vi "Example Circular Buffer Map.vi"() -> ()   [LabVIEW 2013]
uses:
  VariantBuffer/VariantBuffer.lvclass
  VariantBufferMap/VariantBufferMap.lvclass
panel:
  out "last byte":variant
  out "error out":errorcluster
  in  "preview count (-1: all)":i32=5
  out "found":bool
  out "elements":variant[](array[variant])
  in  "Buffer Name":string(combo)
  # "Select the Buffer to Preview"
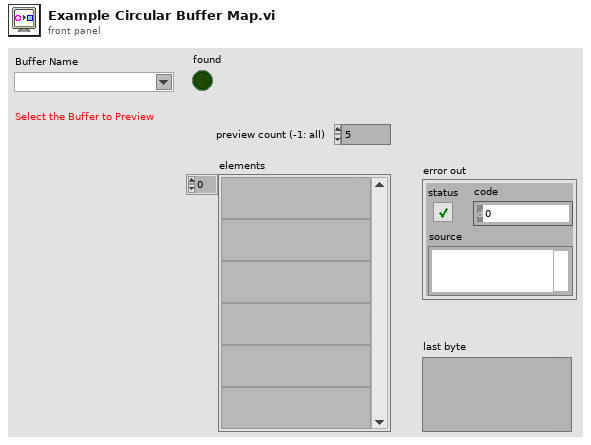
[diagram p1: front panel]
types:
  T1 = typedef "VariantBuffer.lvclass/buffer-event -- enum.ctl" = enum16{"element-added", "element-removed", "filled", "emptied", "resized", "default-changed", "destroyed"}
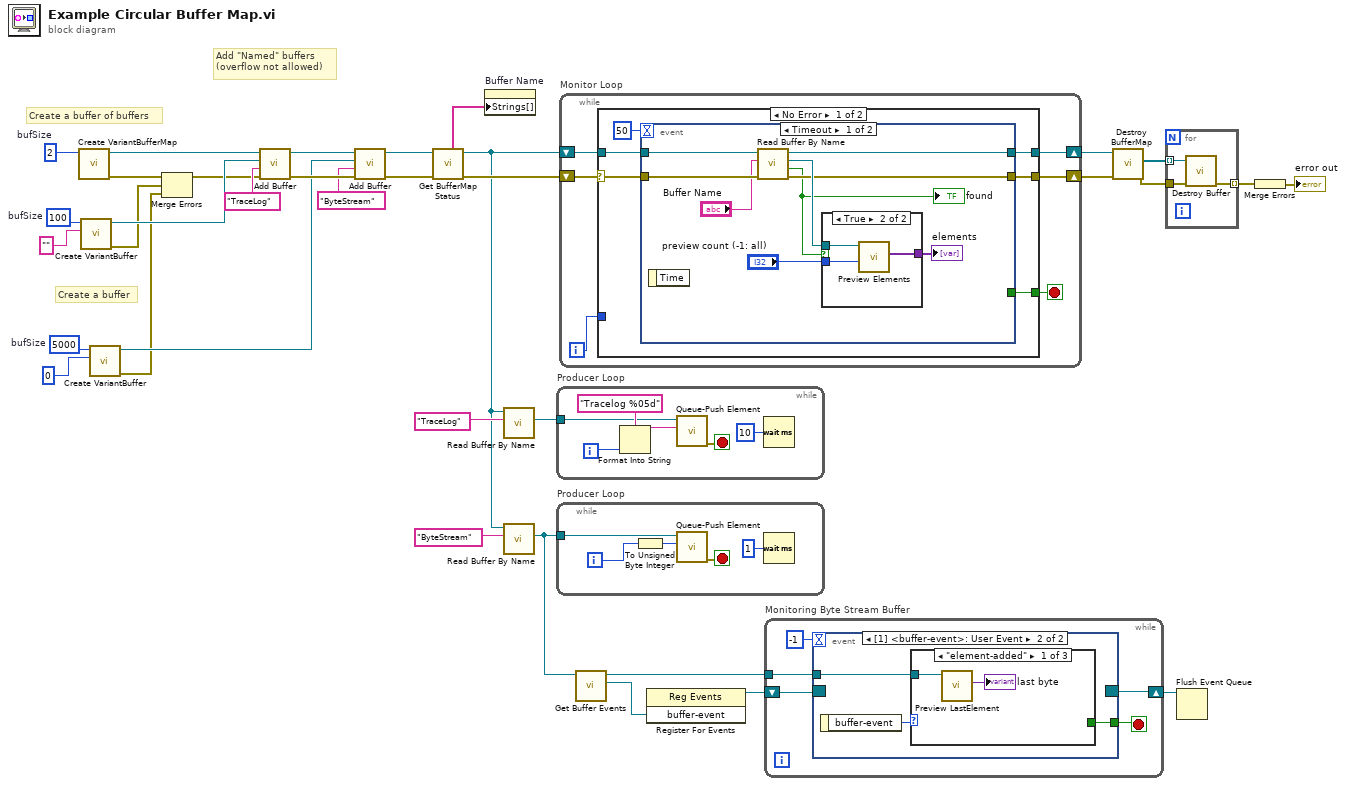
[diagram p0: block diagram]
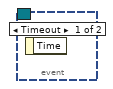
[diagram p2: hidden frame]
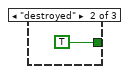
[diagram p3: hidden frame]
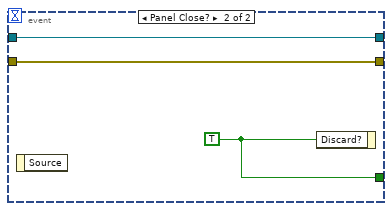
[diagram p6: hidden frame]
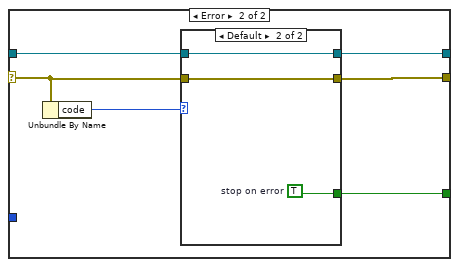
[diagram p7: hidden frame]
diagram:
  w13 = 5000  # bufSize
  w33 = 2  # bufSize
  w35 = 100  # bufSize
  # "Create a buffer"
  # "Add \"Named\" buffers\n(overflow not allowed)"
  # "Create a buffer of buffers"
  n1 = call "Create VariantBufferMap.vi"("bufSize"=w33) -> ("error out"=w26:errorcluster, "BufferMap"=w27:refnum<data-value>)  [unwired: 9 in]
  n2 = call "Create VariantBuffer.vi"("default"="", "bufSize"=w35) -> ("error out"=w25:errorcluster, "Buffer"=w31:refnum<data-value>)  [unwired: 8 in]
  n3 = call "Create VariantBuffer.vi"("default"=u8 0, "bufSize"=w13) -> ("error out"=w9:errorcluster, "Buffer"=w11:refnum<data-value>)  [unwired: 8 in]
  n4 = Merge Errors(w26, w25, w9) -> (w24:errorcluster)
  n5 = call "Add Buffer.vi"("error in"=w24, "Name"="TraceLog", "Buffer"=w31, "BufferMap in"=w27) -> ("error out"=w16:errorcluster, "BufferMap"=w18:refnum<data-value>)  [unwired: 6 in]
  n6 = call "Add Buffer.vi"("error in"=w16, "Name"="ByteStream", "Buffer"=w11, "BufferMap in"=w18) -> ("error out"=w15:errorcluster, "BufferMap"=w17:refnum<data-value>)  [unwired: 6 in]
  n7 = call "Get BufferMap Status.vi"("error in"=w15, "BufferMap in"=w17) -> ("error out"=w21:errorcluster, "BufferMap"=w19:refnum<data-value>, "Names"=w22:string[])  [unwired: 4 in, 3 out]
  n8 = property on="Buffer Name" class="CmbBox"("Strings[]"=w22) -> ()  [unwired: 2 in, 2 out]
  n9 = call "Read Buffer By Name.vi"("Name"="TraceLog", "BufferMap in"=w19) -> ("Buffer"=w28:refnum<data-value>)  [unwired: 6 in, 3 out]
  n10 = call "Read Buffer By Name.vi"("Name"="ByteStream", "BufferMap in"=w19) -> ("Buffer"=w5:refnum<data-value>)  [unwired: 6 in, 3 out]
  n11 = while "Producer Loop" {
    tunnel: w28 -> [w38]
    i -> [w40]
    stop <- w36 stop-if-true
    n12 = Format Into String(format string="Tracelog %05d", w40) -> (resulting string=w37:string)  [unwired: 2 in, 1 out]
    n13 = call "Queue-Push Element.vi"("element"=w37, "Buffer in"=w38) -> ("error out"=w36:errorcluster)  [unwired: 6 in, 3 out]
    n14 = Wait (ms)(milliseconds to wait=u32 10) -> ()  [unwired: 1 out]
  }
  n15 = while "Producer Loop" {
    tunnel: w5 -> [w45]
    i -> [w42]
    stop <- w44 stop-if-true
    n16 = To Unsigned Byte Integer(number=w42) -> (unsigned 8bit integer=w43:u8)
    n17 = call "Queue-Push Element.vi"("element"=w43, "Buffer in"=w45) -> ("error out"=w44:errorcluster)  [unwired: 6 in, 3 out]
    n18 = Wait (ms)(milliseconds to wait=u32 1) -> ()  [unwired: 1 out]
  }
  n19 = while "Monitor Loop" {
    shift-right: [w51] -> w30
    shift-left: w19 -> [w52]
    shift-right: [w50] -> w23
    shift-left: w21 -> [w48]
    i -> [w47]
    stop <- w49 stop-if-true
    n20 = case shown="No Error" w48 {
      selector: w48 -> [w53 w75]
      tunnel: w52 -> [w57 w76]
      tunnel: [w56 w77] -> w51
      tunnel: [w55 w74] -> w50
      tunnel: [w54 w79] -> w49
      tunnel: w47 -> [_ _]
      frame No Error {
        n21 = event shown="[0] Timeout" {
          selector: _ -> [_ _]
          dyn-events: _ -> [_ _]
          timeout: 50 -> [_ _]
          tunnel: w57 -> [w67 w73]
          tunnel: [w66 w73] -> w56
          tunnel: [_ w72] -> w54
          tunnel: w53 -> [w64 w71]
          tunnel: [w63 w71] -> w55
          event Timeout {
            n22 = event-data() -> ()  [unwired: 1 in, 1 out]
            n23 = call "Read Buffer By Name.vi"("error in (no error)"=w64, "Name"="Buffer Name", "BufferMap in"=w67) -> ("error out"=w63:errorcluster, "found"=w61:bool, "Buffer"=w65:refnum<data-value>, "BufferMap"=w66:refnum<data-value>)  [unwired: 5 in]
            "found" <- w61
            n24 = case shown="True" w61 {
              tunnel: w65 -> [_ w70]
              tunnel: [_ w69] -> w60
              tunnel: "preview count (-1: all)" -> [_ w68]
              frame False {
              }
              frame True {
                n25 = call "Preview Elements.vi"("count (-1: all)"=w68, "ByteBuffer in"=w70) -> ("elements"=w69:variant[])  [unwired: 7 in, 2 out]
              }
            }
            "elements" <- w60
          }
          event Panel Close? {
            w72 = TRUE ("Discard?")
            n26 = event-data() -> ()  [unwired: 1 in, 1 out]
            n27 = event-data("Discard?"=w72) -> ()  [unwired: 1 in, 1 out]
          }
        }
      }
      frame Error {
        n28 = Unbundle By Name(w75) -> ("code"=w78:i32)
        n29 = case shown="Default" w78 {
          tunnel: [_ w83] -> w79
          tunnel: [w80 w82] -> w77
          tunnel: w76 -> [w80 w82]
          tunnel: w75 -> [_ w81]
          tunnel: [_ w81] -> w74
          frame 0 {
            # "Handle Error\n& Continue"
          }
          frame Default {
            w83 = TRUE  # stop on error
          }
        }
      }
    }
  }
  n30 = call "Get Buffer Events.vi"("Buffer in"=w5) -> ("buffer-event"=w4:refnum<user-event>, "Buffer"=w2:refnum<data-value>)  [unwired: 8 in, 1 out]
  n31 = register-events(w4) -> (reference out=w3:refnum<event-registration>)  [unwired: 2 in, 1 out]
  n32 = while "Monitoring Byte Stream Buffer" {
    shift-right: [w86] -> w1
    shift-left: w3 -> [w87]
    tunnel: w2 -> [w85]
    stop <- w84 stop-if-true
    n33 = event shown="[1] <buffer-event>: User Event" {
      selector: w87 -> [_ _]
      dyn-events: [_ _] -> w86
      timeout: -1 -> [_ _]
      tunnel: w85 -> [_ w89]
      tunnel: [_ w90] -> w84
      event Timeout {
        n34 = event-data() -> ()  [unwired: 1 in, 1 out]
      }
      event User Event {
        n35 = event-data() -> ("buffer-event"=w91:T1)  [unwired: 1 in]
        n36 = case shown="\"element-added\"" w91 {
          tunnel: [_ TRUE _] -> w90
          tunnel: w89 -> [w93 _ _]
          frame "element-added" {
            n37 = call "Preview LastElement.vi"("Buffer in"=w93) -> ("element"=→"last byte":variant)  [unwired: 7 in, 3 out]
          }
          frame "destroyed" {
          }
          frame Default {
          }
        }
      }
    }
  }
  n38 = call "Destroy BufferMap.vi"("error in"=w23, "Buffer"=w30) -> ("error out"=w8:errorcluster, "elements"=w34:refnum<data-value>[])  [unwired: 8 in]
  n39 = for {
    tunnel: w34 -> [w97] mode=indexing
    tunnel: w8 -> [w96]
    tunnel: [w95] -> w7 mode=indexing
    n40 = call "Destroy Buffer.vi"("error in"=w96, "Buffer"=w97) -> ("error out"=w95:errorcluster)  [unwired: 8 in, 1 out]
  }
  n41 = Flush Event Queue(0:w1) -> ()  [unwired: 5 in, 3 out]
  n42 = Merge Errors(w7) -> (→"error out":errorcluster)
